vi "Rotate First Segment.vi"(9 "Rotated Point":cluster{"x":dbl, "y":dbl, "th":dbl}, 10 "First Segment Point":cluster{"x":dbl, "y":dbl, "th":dbl}, 11 "Original Point":cluster{"x":dbl, "y":dbl, "th":dbl}) -> (3 "New First Segment":cluster{"x":dbl, "y":dbl, "th":dbl})   [LabVIEW 2019]
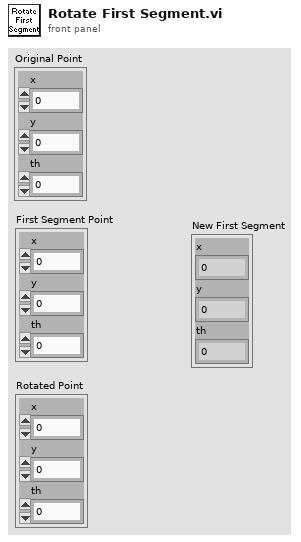
[diagram p1: front panel]
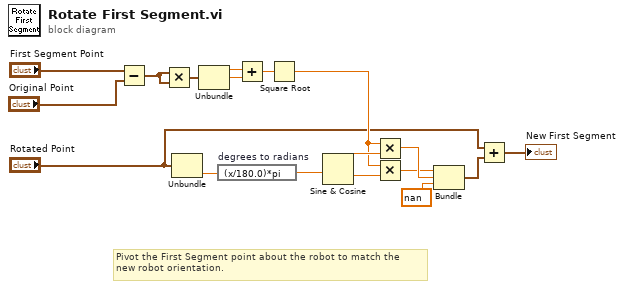
[diagram p0: block diagram]
diagram:
  # "Pivot the First Segment point about the robot to match the\nnew robot orientation."
  n1 = Subtract(x="First Segment Point", y="Original Point") -> (x-y=w16:cluster{"x":dbl, "y":dbl, "th":dbl})
  n2 = Multiply(x=w16, y=w16) -> (x*y=w15:cluster{"x":dbl, "y":dbl, "th":dbl})
  n3 = Unbundle("Rotated Point") -> ("th"=w18:dbl)  [unwired: 2 out]
  n4 = Unbundle(w15) -> ("x"=w14:dbl, "y"=w13:dbl)  [unwired: 1 out]
  n5 = expression code="(x/180.0)*pi" "degrees to radians"(w18) -> (w17:dbl)
  n6 = Add(x=w14, y=w13) -> (x+y=w4:dbl)
  n7 = Square Root(x=w4) -> (sqrt(x)=w3:dbl)
  n8 = Sine & Cosine(0:w17) -> (1:w11:dbl, 2:w12:dbl)
  n9 = Multiply(x=w3, y=w11) -> (x*y=w10:dbl)
  n10 = Multiply(x=w3, y=w12) -> (x*y=w9:dbl)
  n11 = Bundle(w9, w10, nan) -> (w7:cluster{dbl, dbl, dbl})  [unwired: 1 in]
  n12 = Add(x="Rotated Point", y=w7) -> (x+y=→"New First Segment":cluster{dbl, dbl, dbl})
